vi "SimpleGit-SwitchToDailyBranch.vi"(11 "path":path) -> ()   [LabVIEW 2017]
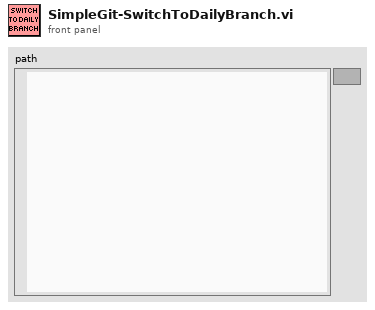
[diagram p1: front panel]
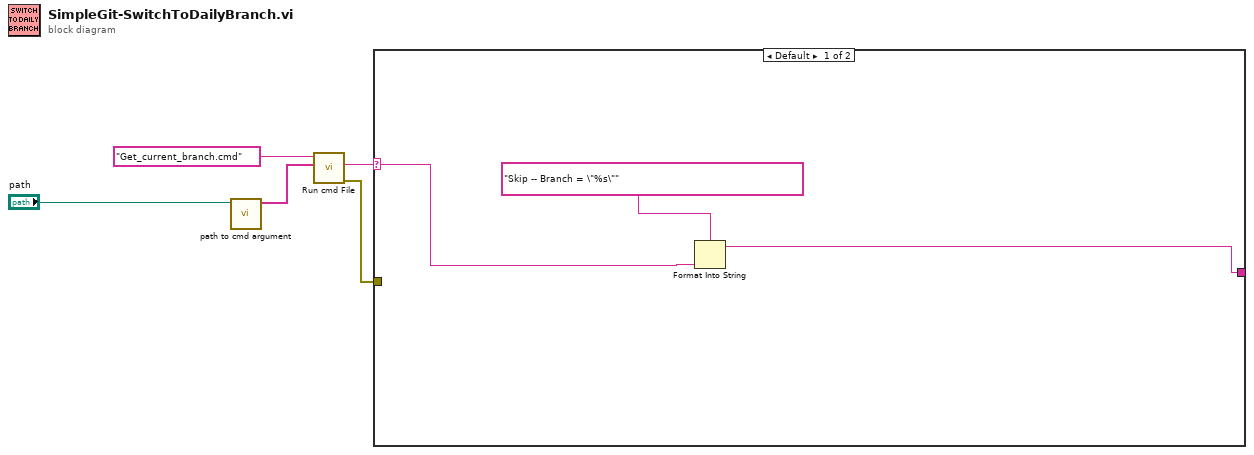
[diagram p0: block diagram]
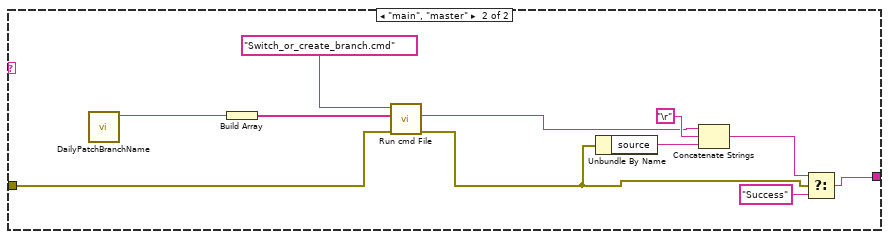
[diagram p2: hidden frame]
diagram:
  n1 = call "path to cmd argument.vi"("path"="path") -> ("Array"=w1:string[])  [unwired: 10 in]
  n2 = call "Run cmd File.vi"("args"=w1, "name or relative path"="Get_current_branch.cmd") -> ("Error out"=w3:errorcluster, "before substring"=w4:string)  [unwired: 7 in, 1 out]
  n3 = case shown="Default" w4 {
    selector: w4 -> [w6 _]
    tunnel: w3 -> [_ w10]
    tunnel: [w7 w15] -> _
    frame Default {
      n4 = Format Into String(format string="Skip -- Branch = \"%s\"" ("f"), w6) -> (resulting string=w7:string)  [unwired: 2 in, 1 out]
    }
    frame "main", "master" {
      n5 = call "DailyPatchBranchName.vi"() -> ("DailyPatchBranchName"=w13:string)  [unwired: 11 in]
      n6 = Build Array(w13) -> (w12:string[])
      n7 = call "Run cmd File.vi"("Error in"=w10, "args"=w12, "name or relative path"="Switch_or_create_branch.cmd") -> ("Error out"=w9:errorcluster, "before substring"=w11:string)  [unwired: 6 in, 1 out]
      n8 = Unbundle By Name(w9) -> ("source"=w18:string)
      n9 = Concatenate Strings(w11, "\r", w18) -> (w19:string)
      n10 = Select(t=w19, s=w9, f="Success") -> (s? t:f=w15:string)
    }
  }
